vi "May Error.vi"   [LabVIEW 2010]
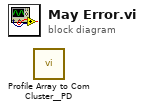
[diagram p0: block diagram]
diagram:
  n1 = call "Profile Array to Com Cluster__PD.vi"() -> ()  [unwired: 1 in, 1 out]
